vi "Serial Decoder.vi"(0 "Write Value":string="108500", 1 "milliseconds to wait":u32=500, 2 "Com Parms":T2={"VISA resource name"="COM6", "baud rate"=38400, "data bits"=8, "parity"=0, "stop bits"=10, "flow control"=0} {"flow control" items=["None"=0, "XON/XOFF"=1, "RTS/CTS"=2, "DTR/DSR"=4]; "stop bits" items=["1.0"=10, "1.5"=15, "2.0"=20]; "parity" items=["None", "Odd", "Even", "Mark", "Space"]; "data bits" min=5 max=8 step=1}, 3 "error in":errorcluster={"status"=FALSE, "code"=-1073807343, "source"=""}) -> (5 "Data Read":T3={"Date"="03/29/13", "Time"="14:47:22", "CO2- ppm"=753, "Last Ctrl Word"=5276928, "O2-1 ppm"=209104, "O2-2 ppm"=209104, "Temp MB"=20.41, "Temp Sensor Modulr"=21.85, "Press mB"=835.52} {"Last Ctrl Word" format="%.0x"}, 7 "error out":errorcluster={"status"=FALSE, "code"=-1073807343, "source"=""})   [LabVIEW 2012]
uses:
  <vilib>/Instr/_visa.llb/VISA Flush IO Buffer Mask.ctl
panel:
  in  "Mask":T1=64 items=["Flush Receive Buffer"=16, "Write Transmit Buffer to Device"=32, "Flush Receive Buffer (No I/O)"=64, "Flush Transmit Buffer"=128]
  out "read buffer":string="03/29/13,14:47:22,753, 00508500, 209104, 209104, 20.41, 21.85, 835.52\r\n"
  out "concatenated string":string="W108500\rR"
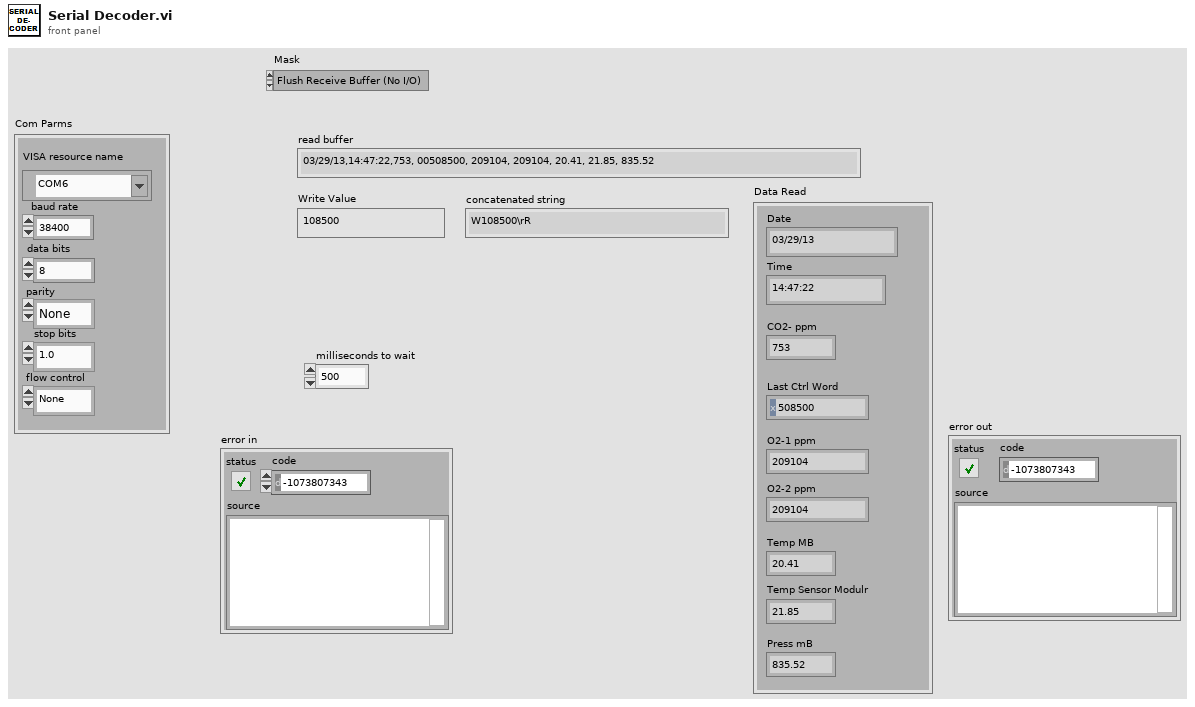
[diagram p1: front panel]
types:
  T1 = typedef "VISA Flush IO Buffer Mask.ctl" = u16
  T2 = cluster{"VISA resource name":refnum<visa-resource-name>, "baud rate":u32, "data bits":u16, "parity":u16, "stop bits":u16, "flow control":u16}
  T3 = cluster{"Date":string, "Time":string, "CO2- ppm":u32, "Last Ctrl Word":u32, "O2-1 ppm":u32, "O2-2 ppm":u32, "Temp MB":sgl, "Temp Sensor Modulr":sgl, "Press mB":sgl}
  T4 = cluster{"default value 1":string, "default value 1":string, "default value 5":u32, "default value 5":u32, "default value 5":u32, "default value 5":u32, "default value 7":sgl, "default value 7":sgl, "default value 7":sgl}
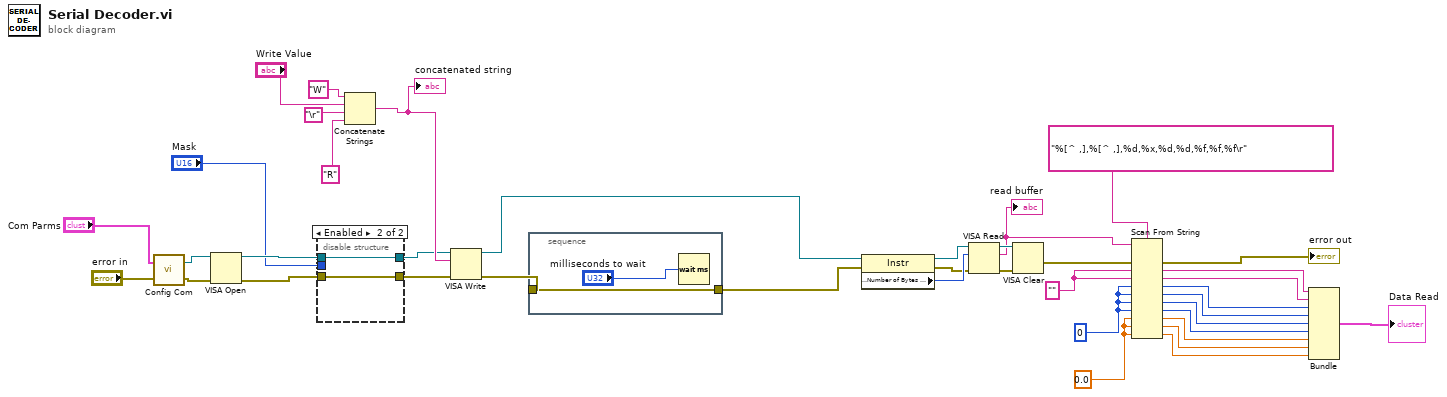
[diagram p0: block diagram]
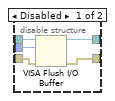
[diagram p2: hidden frame]
diagram:
  w16 = sgl 0.0 ("default value 7")
  w29 = "" ("default value 1")
  w10 = u32 0 ("default value 5")
  n1 = call "Config Com.vi"("error in"="error in", "Com Parms"="Com Parms") -> ("error out"=w14:errorcluster, "VISA resource name out"=w15:refnum<visa-resource-name>)
  n2 = VISA Open(error in (no error)=w14, VISA resource name=w15) -> (VISA resource name=w2:refnum<visa-resource-name>, error out=w5:errorcluster)  [unwired: 3 in]
  n3 = disable-structure shown="Enabled" {
    disable-tunnel: w5 -> [w44 w45]
    disable-tunnel: [w43 w45] -> w4
    disable-tunnel: [w42 w46] -> w3
    disable-tunnel: w2 -> [w41 w46]
    disable-tunnel: "Mask" -> [w40 _]
    frame Disabled {
      n4 = VISA Flush I/O Buffer(VISA resource name=w41, mask (16)=w40, error in (no error)=w44) -> (VISA resource name out=w42:refnum<visa-resource-name>, error out=w43:errorcluster)
    }
    frame Enabled {
    }
  }
  n5 = Concatenate Strings("W" ("string"), "Write Value", "\r", "R" ("string")) -> (w11:string)
  "concatenated string" <- w11
  n6 = VISA Write(VISA resource name=w3, write buffer=w11, error in (no error)=w4) -> (VISA resource name out=w27:refnum<visa-resource-name>, error out=w28:errorcluster)  [unwired: 1 out]
  n7 = stacked-sequence {
    tunnel: [w47] -> w30
    tunnel: w28 -> [w47]
    frame #0 {
      n8 = Wait (ms)(milliseconds to wait="milliseconds to wait") -> ()  [unwired: 1 out]
    }
  }
  n9 = property class="Instr"(reference=w27, error in=w30) -> (reference out=w32:refnum<visa-resource-name>, error out=w31:errorcluster, "Serial Settings:Number of Bytes at Serial Port"=w33:u32)
  n10 = VISA Read(VISA resource name=w32, byte count=w33, error in (no error)=w31) -> (VISA resource name out=w38:refnum<visa-resource-name>, read buffer=w37:string, error out=w36:errorcluster)  [unwired: 1 out]
  "read buffer" <- w37
  n11 = VISA Clear(VISA resource name=w38, error in (no error)=w36) -> (error out=w35:errorcluster)  [unwired: 1 out]
  n12 = Scan From String(format string="%[^ ,],%[^ ,],%d,%x,%d,%d,%f,%f,%f\r" ("String"), input string=w37, error in=w35, default 1=w29, default 2=w29, default 3=w10, default 4=w10, default 5=w10, default 6=w10, default 7=w16, default 8=w16, default 9=w16) -> (error out=→"error out":errorcluster, output 1=w26:string, output 2=w25:string, output 3=w24:u32, output 4=w23:u32, output 5=w22:u32, output 6=w21:u32, output 7=w20:sgl, output 8=w19:sgl, output 9=w18:sgl)  [unwired: 1 in, 2 out]
  n13 = Bundle("default value 1"=w26, "default value 1"=w25, "default value 5"=w24, "default value 5"=w23, "default value 5"=w22, "default value 5"=w21, "default value 7"=w20, "default value 7"=w19, "default value 7"=w18) -> (→"Data Read":T4)  [unwired: 1 in]
